vi "Get Column Definition String.vi"(6 "Column Index (0=Primary Key)":i32, 8 "error in (no error)":errorcluster, 9 "Data Type":T1, 10 "Column Name":string, 11 "PostgreSQL in":refnum<class "PostgreSQL.lvclass">) -> (0 "error out":errorcluster, 1 "Column Definition String":string, 2 "Column Name out":string, 3 "PostgreSQL out":refnum<class "PostgreSQL.lvclass">)   [LabVIEW 2018, in "Database.lvlib" / "PostgreSQL.lvclass"]
uses:
  PostgreSQL.lvclass
  <vilib>/Utility/Data Type/Type Definitions/Data Type.ctl
  <vilib>/Utility/Data Type/NI_Data Type.lvlib
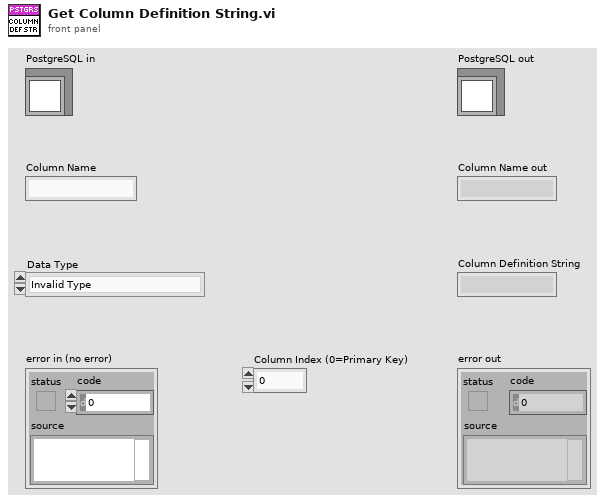
[diagram p1: front panel]
types:
  T1 = typedef "NI_Data Type.lvlib/Data Type.ctl" = enum8{"Invalid Type", "Void", "I8", "I16", "I32", "I64", "U8", "U16", "U32", "U64", "Single Float", "Double Float", "Extended Float", "Single Complex", "Double Complex", "Extended Complex", "Enum U8", "Enum U16", "Enum U32", "Enum U64", "Single Float With Unit", "Double Float With Unit", "Extended Float With Unit", "Single Complex with Unit", "Double Complex with Unit", "Extended Complex with Unit", "Boolean", "String", "Path", "Picture", "Tag", "Array", "Cluster", "Variant", "LV Variant", "Waveform", "Timestamp", "Digital Waveform", "Digital Data", "ExpressData", "Refnum", "External Data", "VI", "Poly VI", "LabVIEW Class Instance", "Fixed Point"}
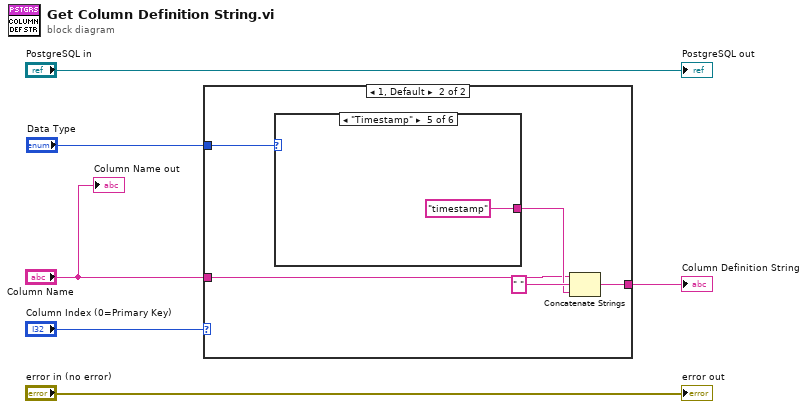
[diagram p0: block diagram]
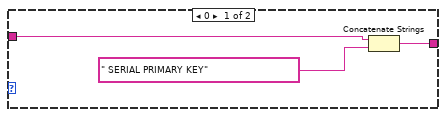
[diagram p2: hidden frame]
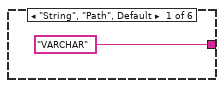
[diagram p3: hidden frame]
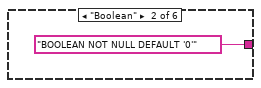
[diagram p4: hidden frame]
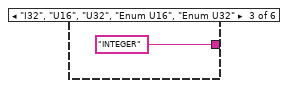
[diagram p5: hidden frame]
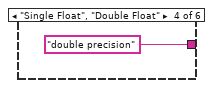
[diagram p6: hidden frame]
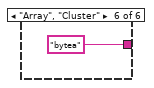
[diagram p7: hidden frame]
diagram:
  n1 = case shown="1, Default" "Column Index (0=Primary Key)" {
    tunnel: "Data Type" -> [_ w14]
    tunnel: "Column Name" -> [w8 w10]
    tunnel: [w9 w11] -> w3
    frame 0 {
      n2 = Concatenate Strings(w8, " SERIAL PRIMARY KEY" ("string")) -> (w9:string)
    }
    frame 1, Default {
      n3 = case shown="\"Timestamp\"" w14 {
        tunnel: ["VARCHAR" ("name") "BOOLEAN NOT NULL DEFAULT '0'" ("name") "INTEGER" ("name") "double precision" ("name") "timestamp" ("name") "bytea" ("name")] -> w12
        frame "String", "Path", Default {
        }
        frame "Boolean" {
        }
        frame "I32", "U16", "U32", "Enum U16", "Enum U32" {
        }
        frame "Single Float", "Double Float" {
        }
        frame "Timestamp" {
        }
        frame "Array", "Cluster" {
        }
      }
      n4 = Concatenate Strings(w10, " " ("string"), w12) -> (w11:string)
    }
  }
  "Column Definition String" <- w3
  "error out" <- "error in (no error)"
  "PostgreSQL out" <- "PostgreSQL in"
  "Column Name out" <- "Column Name"
